vi "Add File Test.vi"() -> ()   [LabVIEW 2018, in "Collaborator.lvlib"]
uses:
  Collaborator.lvlib
  Command Configuration.ctl
  779c1876-450a-4971-bed5-beecc10f443e.vi
  5adfef45-c071-4b71-8614-ee5e75be5eca.vi
  <vilib>/JDP Science/JSONtext/Variant to JSON Text.vi
  Web Client/Web Client.lvclass
  <vilib>/JDP Science/JSONtext/JSONtext.lvlib
panel:
  in  "Review ID":string
  out "<JSON>":string
  in  "File to Add":path
  out "error out":errorcluster
  out "Response":string
  in  "Address":string
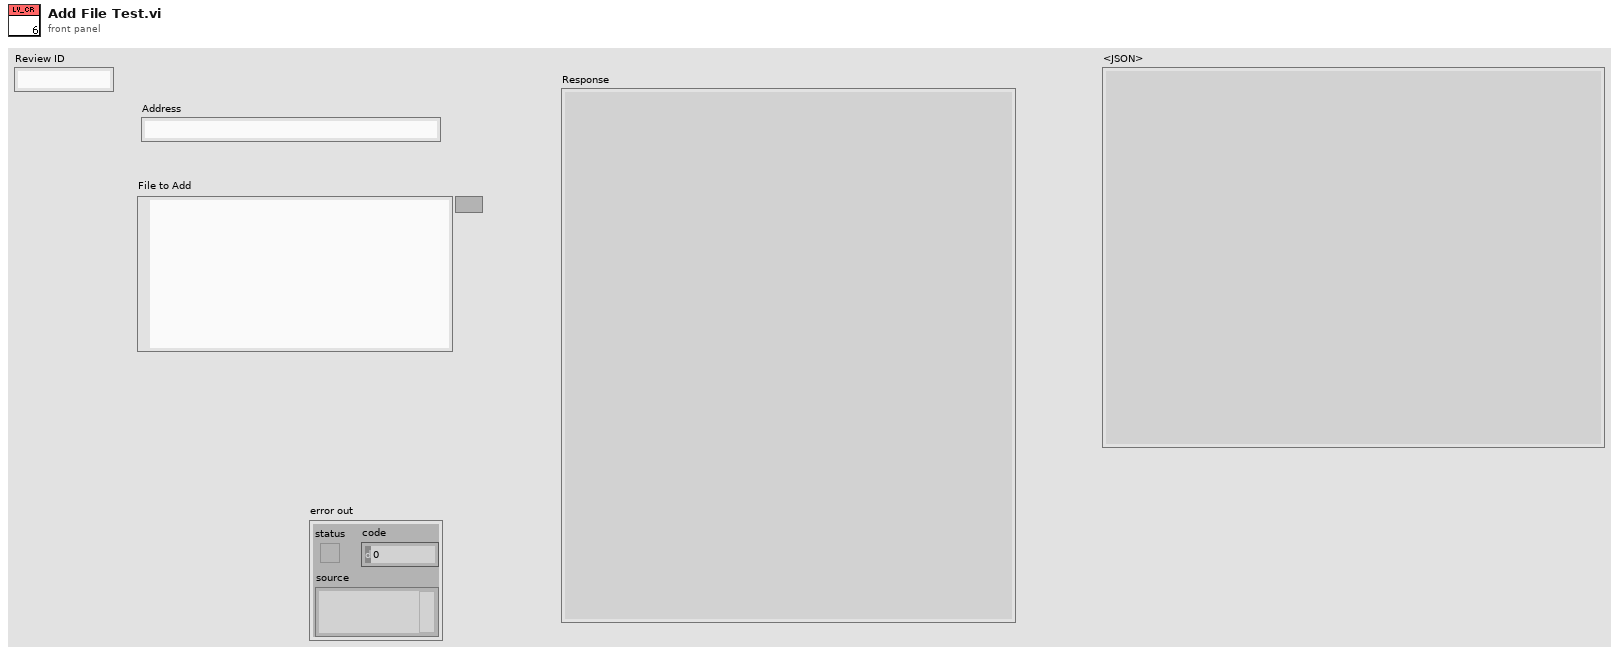
[diagram p1: front panel]
types:
  T1 = typedef "Collaborator.lvlib/Command Configuration.ctl" = cluster{"Interface Name":string, "Method Name":string, "Arguments":cluster{"Argument Name":string, "Argument Value":string}[]}
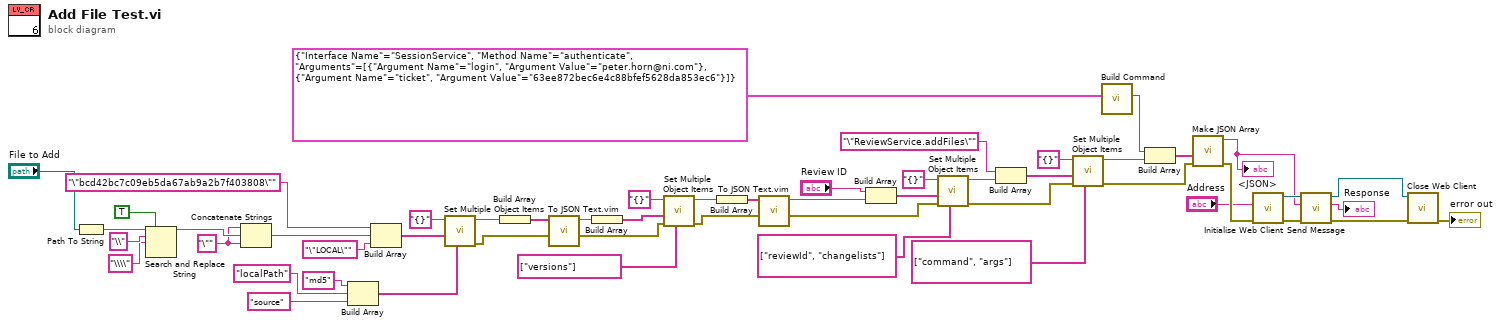
[diagram p0: block diagram]
diagram:
  w42 = "\"" ("string")
  n1 = Path To String(path="File to Add") -> (string=w4:string)
  n2 = Search and Replace String(replace all?=TRUE ("replace all? (F)"), input string=w4, search string="\\", replace string="\\\\" ("replace string (\"\")")) -> (result string=w48:string)  [unwired: 4 in, 3 out]
  n3 = Concatenate Strings(w42, w48, w42) -> (w43:string)
  n4 = Build Array("md5" ("$Path or Item Name"), "localPath" ("$Path or Item Name"), "source" ("element")) -> (w45:string[])
  n5 = Build Array("\"bcd42bc7c09eb5da67ab9a2b7f403808\"" ("element"), w43, "\"LOCAL\"" ("element")) -> (w44:string[])
  n6 = call <vilib>:"Set Multiple Object Items.vi"("Item Names"=w45, "JSON Items"=w44, "JSON"="{}") -> ("error out"=w10:errorcluster, "<JSON>"=w41:string)  [unwired: 6 in]
  n7 = Build Array(w41) -> (w40:string[])
  n8 = call "To JSON Text.vim"("error in (no error)"=w10, "Anything"=w40) -> ("error out"=w9:errorcluster, "<JSON>"=w38:string)  [unwired: 8 in]
  n9 = Build Array(w38) -> (w36:string[])
  n10 = call <vilib>:"Set Multiple Object Items.vi"("Item Names"=string[] ["versions"] ("element"), "error in (no error)"=w9, "JSON Items"=w36, "JSON"="{}") -> ("error out"=w8:errorcluster, "<JSON>"=w33:string)  [unwired: 5 in]
  n11 = Build Array(w33) -> (w32:string[])
  n12 = call "To JSON Text.vim"("error in (no error)"=w8, "Anything"=w32) -> ("error out"=w7:errorcluster, "<JSON>"=w31:string)  [unwired: 8 in]
  n13 = Build Array("Review ID", w31) -> (w28:string[])
  n14 = call <vilib>:"Set Multiple Object Items.vi"("Item Names"=string[] ["reviewId", "changelists"] ("element"), "error in (no error)"=w7, "JSON Items"=w28, "JSON"="{}") -> ("error out"=w6:errorcluster, "<JSON>"=w23:string)  [unwired: 5 in]
  n15 = Build Array("\"ReviewService.addFiles\"" ("element"), w23) -> (w24:string[])
  n16 = call <vilib>:"Set Multiple Object Items.vi"("Item Names"=string[] ["command", "args"] ("$Path or Item Name"), "error in (no error)"=w6, "JSON Items"=w24, "JSON"="{}") -> ("error out"=w5:errorcluster, "<JSON>"=w19:string)  [unwired: 5 in]
  n17 = call "Build Command.vi"("Command Definition"=T1 {"Interface Name"="SessionService", "Method Name"="authenticate", "Arguments"=[{"Argument Name"="login", "Argument Value"="peter.horn@ni.com"}, {"Argument Name"="ticket", "Argument Value"="63ee872bec6e4c88bfef5628da853ec6"}]}) -> ("Command"=w20:string)  [unwired: 10 in]
  n18 = Build Array(w20, w19) -> (w18:string[])
  n19 = call <vilib>:"Make JSON Array.vi"("error in (no error)"=w5, "JSON Elements"=w18) -> ("error out"=w53:errorcluster, "<JSON>"=w1:string)  [unwired: 8 in]
  "<JSON>" <- w1
  n20 = call "Initialise Web Client.vi"("error in (no error)"=w53, "Address"="Address") -> ("error out"=w16:errorcluster, "Web Client out"=w17:refnum<class "Web Client.lvclass">)  [unwired: 8 in]
  n21 = call "Send Message.vi"("error in (no error)"=w16, "Message Data"=w1, "Web Client in"=w17) -> ("error out"=w15:errorcluster, "Response"=→"Response":string, "Web Client out"=w11:refnum<class "Web Client.lvclass">)  [unwired: 6 in]
  n22 = call "Close Web Client.vi"("error in (no error)"=w15, "Web Client in"=w11) -> ("error out"=→"error out":errorcluster)  [unwired: 9 in]
